vi "onthefly2DfitR4_joe.vi"(0 "Detuning in MHz":dbl=3.1200000000000045, 1 "Wavelength (m)":dbl=4.61e-07, 2 "pass image method":bool=TRUE, 3 "Natural Linewidth of Transition\n(ion fwhm in MHz)":dbl=32.0, 4 "Scale Base Level?":bool, 5 "Systematic Broadening in MHz\n(e.g., 3*naturalwidth)":dbl, 6 "Atoms":sgl[][](array[numeric])=array128x160[20480 elements] format="%0.3f", 10 "Background":sgl[][](array[numeric])=array128x160[20480 elements] format="%0.3f", 12 "Specifics of Fitting Routines":T3={"sampleinterleave"=1.0, "pixelsize"=1.04e-05, "CCDbinning"=1.0, "cutborders"=0.0, "number for scale"=5.0, "limit"=5.0, "guesssmoothsize"=1.0}, 18 "Software bin size":dbl=1.0, 19 "Iteration #":i32=17) -> (7 "2-D Gaussian Fit Parameters":T2={"amplitude"=0.8892961577453615, "sigma_y (m)"=0.0010716344200523828, "sigma_x (m)"=0.0011282187646071032, "row offset (pixel #)"=107.09090196307163, "col offset (pixel #)"=64.60863610301513, "offset"=0.0023484310835031282, "slope x"=3.501893060231643e-06, "slope y"=-1.2386464094312888e-05, 0.0}, 8 "opticaldepthimagesingle\n(ln(atoms)-ln(back))(-1)":dbl[][](graph), 9 "peak OD":dbl=0.8892961577453615, 11 "95% confidence intervals":dbl[][](array[numeric])=[[0.8878200954605137, 0.8907722200302094], [12.85779707503883, 12.902645714681908], [13.536711566357582, 13.583931813620858], [107.06932488748916, 107.1124790386541], [64.585796563439, 64.63147564259125], [0.0021145781066604402, 0.0025822840603458162], [-4.1229500025295996e-07, 7.416081120716245e-06], [-1.707838635719088e-05, -7.694541831434894e-06]], 13 "smoothed OD-fit OD":dbl[][](graph), 14 "# atoms from peakOD":dbl=69475747.95013615 format="%#_6e", 15 "# atoms from \nODintegral":dbl=69475747.95013615, 16 "Chi-squared":dbl=4.589730734027751 format="%#_3g", 17 "alpha":dbl=9.775419954480679e-14)   [LabVIEW 2013]
uses:
  <vilib>/Utility/file.llb/Read From Spreadsheet File (DBL).vi
  <vilib>/Analysis/NI_AALPro.lvlib
panel:
  out "2-D Array of Real":dbl[][](array[numeric])
  in  "Case Constant\n(See Context Help) 3":bool=TRUE
  in  "Case Constant\n(See Context Help) 2":bool=TRUE
  in  "Case Constant\n(See Context Help)":bool
  in  "Read from Binary?":bool=TRUE
  out "Atoms 2":sgl[][](array[numeric])
  out "min index(es)":i32[](array[numeric])=[114, 65]
  out "min value":sgl=98108.0
  out "max index(es)":i32[](array[numeric])=[57, 62]
  out "max value":sgl=690763.0
  out "size(s)":i32[](array[numeric])=[160, 128]
  out "ROI (no binning)":sgl[][](graph)
  out "max indices on\noutput image":i32[](array[numeric])=[96, 56]
  in  "Cut image?":bool
  in  "ROI Controls":T1={"row index"=110, "# rows"=440, "col index"=600, "# cols"=550}
  out "peak indices on\ninput image":i32[](array[numeric])=[96, 56]
  out "error out":errorcluster
  in  "saved image dimensions\n(if saved file is binary)":i32[](array[numeric])=[1024, 1280]
  in  "File Path for image (not background)":path=path "C:/instrumentvi/development/2dfits/20050818atomstestfitB.bny"
  in  "File Path for electronic\nbackground image (must be\nsame size as image of atoms)":path=path "C:/instrumentvi/development/2dfits/20050818backtestfitB.bny"
  out "smoothed optical depth":dbl[][](graph)
  out "fit optical depth":dbl[][](graph)
  out "Background":dbl[][](graph)
  out "Atoms":dbl[][](graph)
  # "Can be gotten\nfrom batch file"
  # "number of columns and rows to scale the base level of atom and background images"
  # "(total column size in each data file should be an integer multiple of sampleinterleave) for big matrices form a matrix using only one point for every sampleinterleave points in a row/column"
  # "the real size for the object in meter unit for a pixel"
  # "number of columns and rows at the corners to find the uncertainities/noise"
  # "total binning"
  # "(REMEMBER THIS IS DONE AFTER SAMPLEINTERLEAVE) number of columns and rows to trim on either side of the data matrix"
  # "number of pixels in smoothing for plotting residuals"
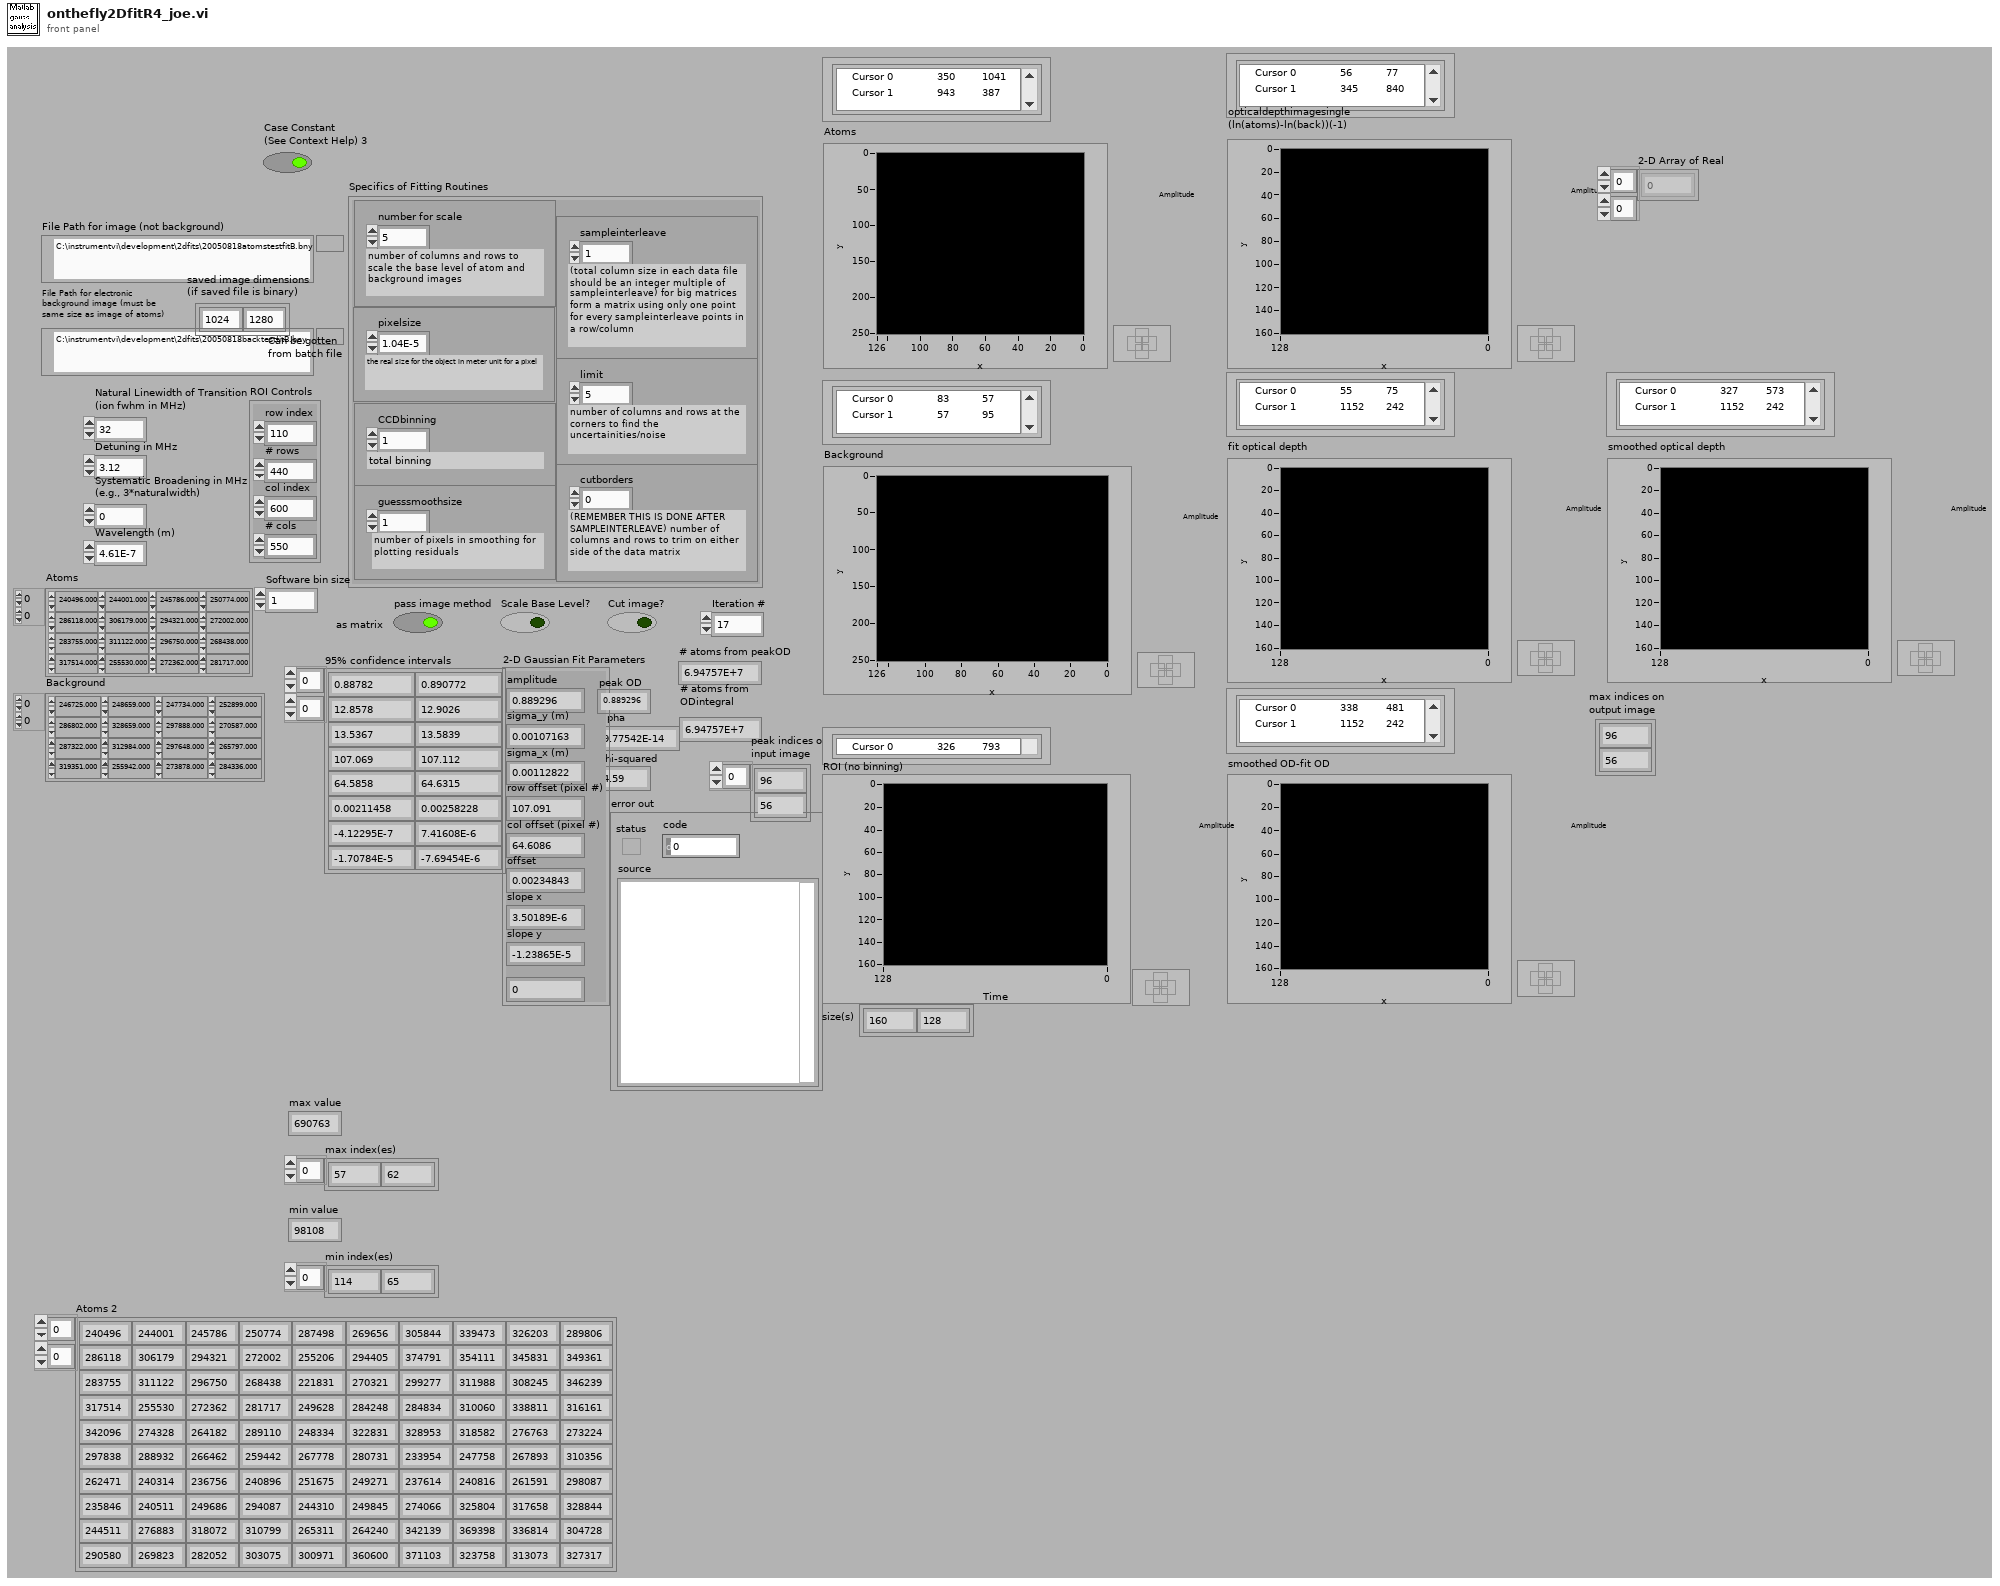
[diagram p1: front panel]
types:
  T1 = cluster{"row index":i32, "# rows":i32, "col index":i32, "# cols":i32}
  T2 = cluster{"amplitude":dbl, "sigma_y (m)":dbl, "sigma_x (m)":dbl, "row offset (pixel #)":dbl, "col offset (pixel #)":dbl, "offset":dbl, "slope x":dbl, "slope y":dbl, dbl}
  T3 = cluster{"sampleinterleave":dbl, "pixelsize":dbl, "CCDbinning":dbl, "cutborders":dbl, "number for scale":dbl, "limit":dbl, "guesssmoothsize":dbl}
  T4 = cluster{"[0]":dbl, "[1]":dbl, "[2]":dbl, "[3]":dbl, "[4]":dbl, "[5]":dbl, "[6]":dbl, "[7]":dbl, "[8]":dbl}
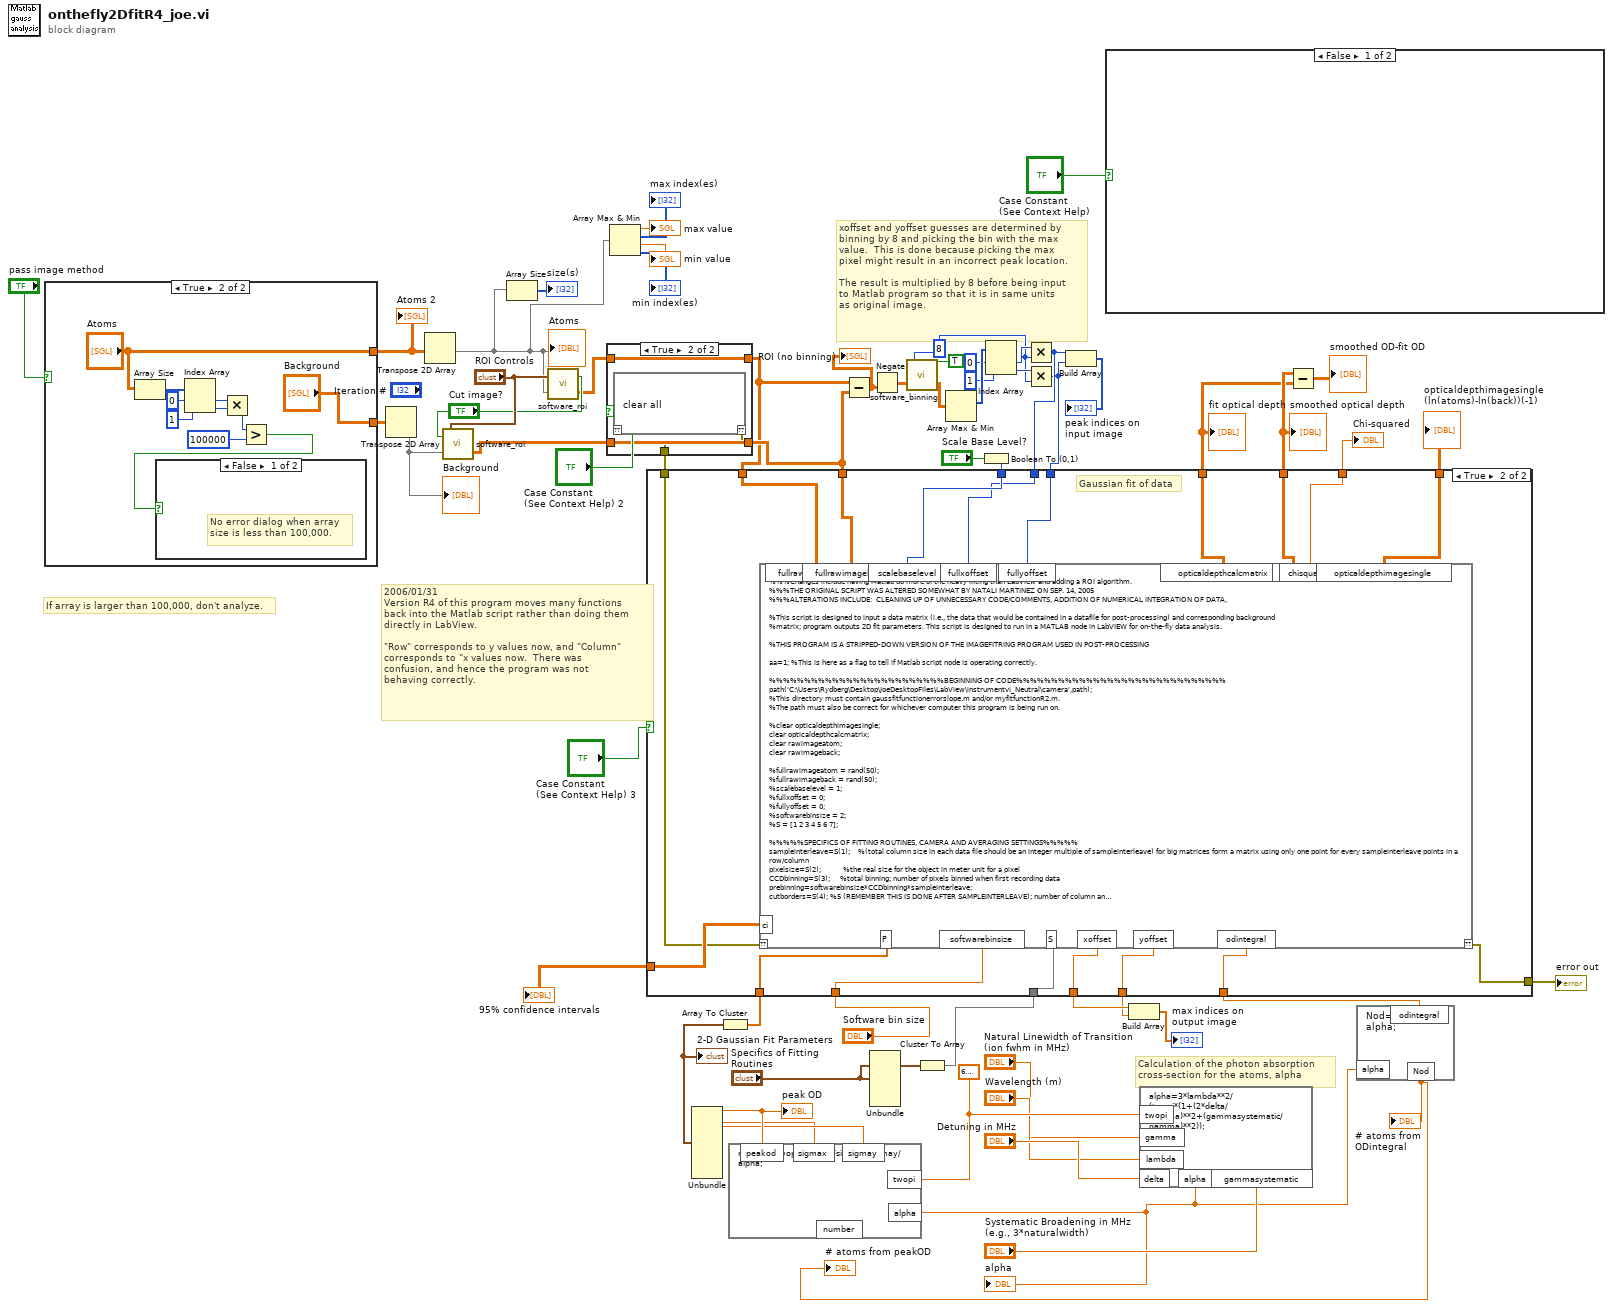
[diagram p0: block diagram]
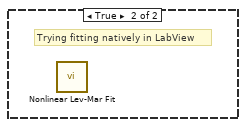
[diagram p2: hidden frame]
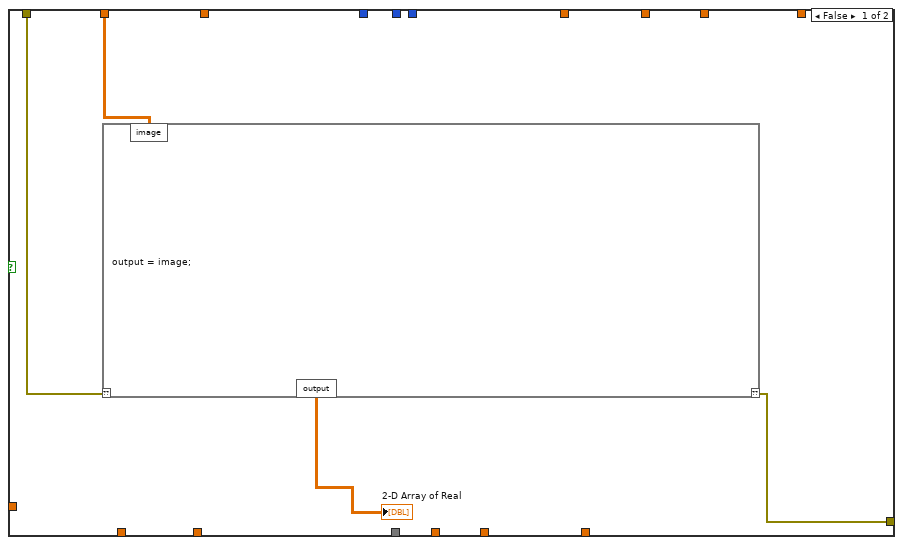
[diagram p3: hidden frame]
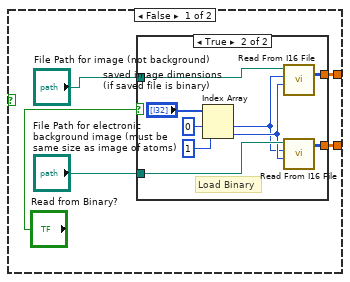
[diagram p5: hidden frame]
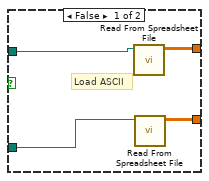
[diagram p6: hidden frame]
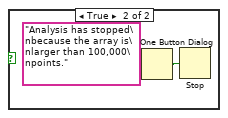
[diagram p7: hidden frame]
diagram:
  w39 = 8 ("bin size")
  w61 = 6.283185307179586
  # "If array is larger than 100,000, don't analyze."
  # "2006/01/31\nVersion R4 of this program moves many functions\nback into the Matlab script rather than doing them\ndirectly in LabView.\n\n\"Row\" corresponds to y values now, and \"Column\"\ncorresponds to \"x values now.  There was\nconfusion, and hence the program was not\nbehaving correctly."
  # "xoffset and yoffset guesses are determined by\nbinning by 8 and picking the bin with the max\nvalue.  This is done because picking the max\npixel might result in an incorrect peak location.\n\nThe result is multiplied by 8 before being input\nto Matlab program so that it is in same units\nas original image."
  # "Calculation of the photon absorption\ncross-section for the atoms, alpha"
  n1 = case shown="True" "pass image method" {
    tunnel: [w66 "Atoms"] -> w16
    tunnel: [w65 "Background"] -> w15
    frame False {
      n2 = case shown="True" "Read from Binary?" {
        tunnel: [w70 w79] -> w66
        tunnel: [w69 w78] -> w65
        tunnel: "File Path for image (not background)" -> [w68 w76]
        tunnel: "File Path for electronic\nbackground image (must be\nsame size as image of atoms)" -> [w67 w77]
        frame False {
          # "Load ASCII"
          n3 = call-poly <vilib>:"Read From Spreadsheet File.vi"("file path (dialog if empty)"=w68) -> ("all rows"=w70:dbl[][])  [unwired: 6 in, 4 out]
          n4 = call-poly <vilib>:"Read From Spreadsheet File.vi"("file path (dialog if empty)"=w67) -> ("all rows"=w69:dbl[][])  [unwired: 6 in, 4 out]
        }
        frame True {
          # "Load Binary"
          n5 = Index Array(array="saved image dimensions\n(if saved file is binary)", index #1=0, index #2=1) -> (element #1=w71:i32, element #2=w72:i32)
          n6 = call <vilib>:"Read From I16 File.vi"("2D number of columns/1D count (all as 1D:-1)"=w72, "2D number of rows"=w71, "file path (dialog if empty)"=w76) -> ("2D array"=w79:i16[][])  [unwired: 4 in, 4 out]
          n7 = call <vilib>:"Read From I16 File.vi"("2D number of columns/1D count (all as 1D:-1)"=w72, "2D number of rows"=w71, "file path (dialog if empty)"=w77) -> ("2D array"=w78:i16[][])  [unwired: 4 in, 4 out]
        }
      }
    }
    frame True {
      n8 = Array Size(array="Atoms") -> (size(s)=w87:i32[])
      n9 = Index Array(array=w87, index #1=0 ("index"), index #2=1 ("index")) -> (element #1=w84:i32, element #2=w83:i32)
      n10 = Multiply(x=w84, y=w83) -> (x*y=w82:i32)
      n11 = Greater?(x=w82, y=100000) -> (0:w80:bool)
      n12 = case shown="False" w80 {
        frame False {
          # "No error dialog when array\nsize is less than 100,000."
        }
        frame True {
          n13 = One Button Dialog(message="Analysis has stopped\nbecause the array is\nlarger than 100,000\npoints.") -> (true=w90:bool)  [unwired: 1 in]
          n14 = Stop(stop? (T)=w90) -> ()
        }
      }
    }
  }
  "Atoms 2" <- w16
  n15 = Transpose 2D Array(2D array=w15) -> (transposed array=w13:dbl[][])
  "Background" <- w13
  n16 = Transpose 2D Array(2D array=w16) -> (transposed array=w10:dbl[][])
  "Atoms" <- w10
  n17 = call "software_roi.vi"("Cut image?"="Cut image?", "Input Array"=w13, "ROI Controls"="ROI Controls") -> ("output array"=w12:sgl[][])
  n18 = Array Size(array=w10) -> (size(s)=→"size(s)":i32[])
  n19 = call "software_roi.vi"("Cut image?"="Cut image?", "Input Array"=w10, "ROI Controls"="ROI Controls") -> ("output array"=w14:sgl[][])
  n20 = case shown="True" "Case Constant\n(See Context Help) 2" {
    tunnel: w14 -> [w93 w96]
    tunnel: [w93 w96] -> w25
    tunnel: [w92 w95] -> w26
    tunnel: w12 -> [w92 w95]
    tunnel: [_ w94] -> w11
    frame False {
    }
    frame True {
      n21 = script code="clear all"() -> ("??"=w94:errorcluster)  [unwired: 1 in]
    }
  }
  n22 = Array Max & Min(array=w10) -> (max value=→"max value":dbl, max index (indices)=→"max index(es)":i32[], min value=→"min value":dbl, min index (indices)=→"min index(es)":i32[])
  n23 = Subtract(x=w25, y=w26) -> (x-y=w18:sgl[][])
  "ROI (no binning)" <- w18
  n24 = Unbundle("Specifics of Fitting Routines") -> ()  [unwired: 7 out]
  n25 = Negate(x=w18) -> (-x=w24:sgl[][])
  n26 = call "software_binning.vi"("Bin image?"=TRUE, "Input Array"=w24, "bin size"=w39) -> ("Binned Array"=w32:dbl[][])
  n27 = Cluster To Array(cluster="Specifics of Fitting Routines") -> (array=w3:dbl[])
  n28 = Array Max & Min(array=w32) -> (max index (indices)=w44:i32[])  [unwired: 3 out]
  n29 = Boolean To (0,1)(Boolean="Scale Base Level?") -> (0, 1=w28:i16)
  n30 = Index Array(array=w44, index #1=0 ("index"), index #2=1 ("index")) -> (element #1=w41:i32, element #2=w40:i32)
  n31 = Multiply(x=w41, y=w39) -> (x*y=w23:i32)
  n32 = Multiply(x=w40, y=w39) -> (x*y=w22:i32)
  n33 = case shown="True" "Case Constant\n(See Context Help) 3" {
    tunnel: [_ w103] -> w60
    tunnel: [_ w109] -> w59
    tunnel: [_ w112] -> w57
    tunnel: [_ w104] -> w48
    tunnel: [w100 w110] -> w1
    tunnel: w25 -> [w98 w102]
    tunnel: w26 -> [_ w118]
    tunnel: [_ w111] -> w27
    tunnel: [_ w114] -> w34
    tunnel: [_ w113] -> w35
    tunnel: w28 -> [_ w117]
    tunnel: w23 -> [_ w116]
    tunnel: w22 -> [_ w115]
    tunnel: [_ w106] -> w21
    tunnel: [_ w105] -> w20
    tunnel: w11 -> [w99 w101]
    tunnel: w3 -> [_ w107]
    tunnel: "Software bin size" -> [_ w108]
    frame False {
      n34 = script code="output = image;"("??"=w99, "image"=w98) -> ("??"=w100:errorcluster, "output"=→"2-D Array of Real":dbl[][])
    }
    frame True {
      # "Gaussian fit of data"
      n35 = script code="%%%Last revision 2006/01/30, by Pascal.\n%%%Changes include having Matlab do more of the heavy lifting than LabView and adding a ROI algorithm.\n%%%THE ORIGINAL SCRIPT WAS ALTERED SOMEWHAT BY NATALI MARTINEZ ON SEP. 14, 2005\n%%%ALTERATIONS INCLUDE:  CLEANING UP OF UNNECESSARY CODE/COMMENTS, ADDITION OF NUMERICAL INTEGRATION OF DATA,  \n\n%This script is designed to input a data matrix (i.e., the data that would be contained in a datafile for post-processing) and corresponding background \n%matrix; program outputs 2D fit parameters. This script is designed to run in a MATLAB node in LabVIEW for on-the-fly data analysis.\n\n%THIS PROGRAM IS A STRIPPED-DOWN VERSION OF THE IMAGEFITRING PROGRAM USED IN POST-PROCESSING\n\naa=1; %This is here as a flag to tell if Matlab script node is operating correctly.\n\n%%%%%%%%%%%%%%%%%%%%%%%%%BEGINNING OF CODE%%%%%%%%%%%%%%%%%%%%%%%%%%%%%%\npath('C:\\Users\\Rydberg\\Desktop\\JoeDesktopFiles\\LabView\\instrumentvi_Neutral\\camera',path);\n%This directory must contain gaussfitfunctionerrorslope.m and/or myfitfunctionR2.m.\n%The path must also be correct for whichever computer this program is being run on.\n\n%clear opticaldepthimagesingle;\nclear opticaldepthcalcmatrix;\nclear rawimageatom;\nclear rawimageback;\n\n%fullrawimageatom = rand(50);\n%fullrawimageback = rand(50);\n%scalebaselevel = 1;\n%fullxoffset = 0;\n%fullyoffset = 0;\n%softwarebinsize = 2;\n%S = [1 2 3 4 5 6 7];\n\n%%%%%SPECIFICS OF FITTING ROUTINES, CAMERA AND AVERAGING SETTINGS%%%%%\nsampleinterleave=S(1);    %(total column size in each data file should be an integer multiple of sampleinterleave) for big matrices form a matrix using only one point for every sampleinterleave points in a row/column\npixelsize=S(2);           %the real size for the object in meter unit for a pixel\nCCDbinning=S(3);     %total binning; number of pixels binned when first recording data\nprebinning=softwarebinsize*CCDbinning*sampleinterleave;\ncutborders=S(4); %5 (REMEMBER THIS IS DONE AFTER SAMPLEINTERLEAVE); number of column and rows to trim on either side of the data matrix\nnumberforscale=S(5);     %number of column and rows to scale the base level of atom and background images\nlimit=S(6);     %number of column and rows at the corners to find the uncertainities/noise\nguesssmoothsize=S(7);  %number of points to average for guessing\n\nf=fullrawimageatom;\nfullsizefull=size(fullrawimageatom);\nfullrowfull=fullsizefull(1); %no. of rows; form matrix from only part of the data\nfullcolumnfull=fullsizefull(2);\n\n%%%SCALING OF BASE LEVEL%%%\nif scalebaselevel==1\n     sumylowxlow=sum(sum(fullrawimageatom(1:numberforscale,1:numberforscale)));;\n     sumylowxhigh=sum(sum(fullrawimageatom(1:numberforscale,fullcolumnfull-numberforscale:fullcolumnfull)));\n     sumyhighxlow=sum(sum(fullrawimageatom(fullrowfull-numberforscale:fullrowfull,1:numberforscale)));\n     sumyhighxhigh=sum(sum(fullrawimageatom(fullrowfull-numberforscale:fullrowfull,fullcolumnfull-numberforscale:fullcolumnfull)));\n     baselevelatom=sumylowxlow+sumylowxhigh+sumyhighxlow+sumyhighxhigh;\n     sumylowxlow=sum(sum(fullrawimageback(1:numberforscale,1:numberforscale))); %there was an error I think so changed from average to sum since \n     sumylowxhigh=sum(sum(fullrawimageback(1:numberforscale,fullcolumnfull-numberforscale:fullcolumnfull)));\n     sumyhighxlow=sum(sum(fullrawimageback(fullrowfull-numberforscale:fullrowfull,1:numberforscale)));\n     sumyhighxhigh=sum(sum(fullrawimageback(fullrowfull-numberforscale:fullrowfull,fullcolumnfull-numberforscale:fullcolumnfull)));\n     baselevelback=sumylowxlow+sumylowxhigh+sumyhighxlow+sumyhighxhigh;\n     fullrawimageatom=fullrawimageatom*baselevelback/baselevelatom;\nend\n\n%%%INTERLEAVING OF DATA%%%;  uses every sampleinterleave points and throws away rest of data\ni=0; j=0; v=0;\nfor i=1:fullrowfull/sampleinterleave\n    for j=1:fullcolumnfull/sampleinterleave\n        for v=1:sampleinterleave\n            temp1(v)=sum(fullrawimageatom(((i-1)*sampleinterleave+1):i*sampleinterleave,((j-1)*sampleinterleave+v))); %this does the software interleaving/sampling\n            temp2(v)=sum(fullrawimageback(((i-1)*sampleinterleave+1):i*sampleinterleave,((j-1)*sampleinterleave+v))); %interleaving for background\n        end\n        rawimageatom(i,j)=sum(temp1); %stores the software interleaved/sampled data\n        rawimageback(i,j)=sum(temp2); %stores the software interleaved/sampled data\n    end\nend\nsizefull=size(rawimageatom);\nrowfull=sizefull(1);       %number of rows after interleaving\ncolumnfull=sizefull(2); %number of columns after interleaving\nxoffsetfull=fullxoffset/sampleinterleave; %adjust peak position to new size\nyoffsetfull=fullyoffset/sampleinterleave; %adjust peak position to new size\n\n%%%CUT DATA OFF FROM EDGES%%%; remember this is done after interleaving\ni=0; j=0;\nfor i=1+cutborders:rowfull-cutborders,\n    for j=1+cutborders:columnfull-cutborders,\n        cutimageatom(i-cutborders,j-cutborders)=rawimageatom(i,j);\n        cutimageback(i-cutborders,j-cutborders)=rawimageback(i,j);\n    end\nend\nsizes=size(cutimageatom);\nrow=sizes(1); %number of rows after cutting data off of edges\ncolumn=sizes(2); %number of columns after cutting data off of edges\nxoffset=xoffsetfull-cutborders; %Determines guess for peak position\nyoffset=yoffsetfull-cutborders; %Determines guess for peak position\n\n%%%ABS VALUE AND OPTICAL DEPTH%%%\ncutimageatom=abs(cutimageatom);   %abs gives the absolute value and complex magnitude\ncutimageback=abs(cutimageback);\nopticaldepthimagesingle=(log(cutimageatom)-log(cutimageback))*(-1); %makes absorption positive\n\n%%%DATA FITTING - 2D FITS%%%\n%GENERATE GUESSES AND BOUNDS%\nZguess=filter2(ones(guesssmoothsize,guesssmoothsize),opticaldepthimagesingle(:,:))/guesssmoothsize^2; %atom-back/OD, smoothed for finding guesses   \namplitude=max(max(Zguess));     %this will give trouble if slope is too big\nsigx=column/10;\nsigy=row/10;\n%xoffset=row/2; %xoffset is now input from LabView; determined by binning by 8 and choosing max bin rather than max pixel.\n%yoffset=column/2; %same comment for yoffset as for xoffset.\naverageylowxlow=sum(sum(Zguess(1:5,1:5)))/25;;\naverageylowxhigh=sum(sum(Zguess(1:5,column-5:column)))/25;\naverageyhighxlow=sum(sum(Zguess(row-5:row,1:5)))/25;\naverageyhighxhigh=sum(sum(Zguess(row-5:row,column-5:column)))/25;\noffset=(averageylowxlow+averageylowxhigh+averageyhighxlow+averageyhighxhigh)/4 ;\nslopex=((averageylowxhigh+averageyhighxhigh)-(averageylowxlow+averageyhighxlow))/(2*column);\nslopey=((averageyhighxlow+averageyhighxhigh)-(averageylowxlow+averageylowxhigh))/(2*row);\n     \nInitialConditions=[amplitude, sigx, sigy, xoffset, yoffset,offset,slopex,slopey];\n%lowerbound=[0, 1, 1, 10, 10, -3, 0, 0,-.01,-.01];\n%upperbound=[1, 50, 50, 90, 90, 3, 1, 1,.01,.01];\ntemp5=size(InitialConditions);\nnumberofparameters=temp5(2); %number of 2D fit parameters\n \n%%%STATISTICS OF IMAGE%%%\n%Weird things happen when you calculate these with smoothed images!!!\n%get estimate of noise, you need to subtract image from background because of fringes and variations in intensity\naverage1=sum(sum(cutimageatom(1:limit,1:limit)-cutimageback(1:limit,1:limit)))/limit^2;\nrms1=sqrt(sum(sum((cutimageatom(1:limit,1:limit)-cutimageback(1:limit,1:limit)).^2))/limit^2);\nrmsdeviation1=sqrt(rms1^2-average1^2);\n   \naverage2=sum(sum(cutimageatom(row-limit:row,1:limit)-cutimageback(row-limit:row,1:limit)))/limit^2;\nrms2=sqrt(sum(sum((cutimageatom(row-limit:row,1:limit)-cutimageback(row-limit:row,1:limit)).^2))/limit^2);\nrmsdeviation2=sqrt(rms2^2-average2^2);\n   \naverage3=sum(sum(cutimageatom(1:limit,column-limit:column)-cutimageback(1:limit,column-limit:column)))/limit^2;\nrms3=sqrt(sum(sum((cutimageatom(1:limit,column-limit:column)-cutimageback(1:limit,column-limit:column)).^2))/limit^2);\nrmsdeviation3=sqrt(rms3^2-average3^2);\n\naverage4=sum(sum(cutimageatom(row-limit:row,column-limit:column)-cutimageback(row-limit:row,column-limit:column)))/limit^2;\nrms4=sqrt(sum(sum((cutimageatom(row-limit:row,column-limit:column)-cutimageback(row-limit:row,column-limit:column)).^2))/limit^2);\nrmsdeviation4=sqrt(rms4^2-average4^2);\n   \nerror=abs((rmsdeviation1+rmsdeviation2+rmsdeviation3+rmsdeviation4)/(4))\n\n%%%CREATE FITTING MATRICES%%%\n%SEE EXPLANATION ON PG. 78 OF PRIYA'S NOTEBOOK 2 %\nerrorod(1:row*column)=error/(sum(sum(cutimageback))/(row*column));     %normalized error - relative to average pixel value\nxvec=1:column;\nyvec=1:row;\n[ydata,xdata]=meshgrid(yvec,xvec);     %rows of output array xdata are copies of vector xvec; columns of output array ydata are copies of vector yvec\nydata=transpose(ydata); xdata=transpose(xdata);\nnumberofpoints=column*row*ones(column,row);     %matrix in which each entry is the number of points \ncoordmatrix=[ydata(:),xdata(:),errorod(:),numberofpoints(:)];\n \n%%%ACTUAL FITTING PROCEDURES%%%  \nZ2=(opticaldepthimagesingle(:)./(errorod(:)*sqrt(column*row)));     %flattened(1D) list of image weighted by uncertainties, not smoothed\noptions=statset('MaxIter',12);\n\n%%%nlinfit method%%%\n[P,r,J,iteractual]=nlinfit(coordmatrix,Z2(:),@gaussfitfunctionerrorsslope,InitialConditions,options);     % expecting data divided by weight and sqrt(number of points)\n\n%%%Gauss-Newton least squares%%%\n%maxiter = 10;\n%tol = 10e-5;\n%P = InitialConditions';\n    %for iter = 1:maxiter\n        %[r,J] = feval(@myfitfunctionR2,P,coordmatrix,Z2);\n        %g = J'*r;\n        %nrmg = norm(g);\n        %fprintf('iter: %2i  norm(g) = %7.3e\\n',iter,nrmg);\n        %if nrmg < tol break; end\n\n        %f = 0.5*r'*r;\n        %B = J'*J+min(10e-4,2*f)*speye(size(J,2));\n        %P = P - B\\g;\n    %end\n%P=P';\n\n%%%REMOVE THE GRADIENT FROM THE DATA%%% ; that is, remove background and slope from data\ngradmatrix=(ydata(:)-P(5))*P(8)+(xdata(:)-P(4))*P(7)+P(6);\nnogradoddata=opticaldepthimagesingle(:)-gradmatrix(:);\nnogradodmatrix = reshape(nogradoddata, size(ydata));  %returns an n-dimensional array with same elements as nograddata but reshaped to size(ydata)\n\n%%%Generate plot of optical density based on fitted parameters, remove distortion of data due to dividing by weight and sqrt(number of points)%%%\ndummyerrorod(1:row*column)=1; \ndummynumberofpoints=ones(row,column); \ncoordmatrix=[ydata(:),xdata(:),dummyerrorod(:),dummynumberofpoints(:)];\nopticaldepthcalcvector=gaussfitfunctionerrorsslope(P, coordmatrix);     %optical depth calculated from fit paramters\nopticaldepthcalcmatrix=reshape(opticaldepthcalcvector,size(ydata));\n\nci=nlparci(P,r,J);%error in the fit parameters 95% confidence interval\nsdev=(ci(:,2)-ci(:,1))/4;%turn confidence interval into 1 sigma             \nweightedresidue3D=(Z2(:)-gaussfitfunctionerrorsslope(P, coordmatrix)); %weighted residues\nchi3D=(transpose(weightedresidue3D)*weightedresidue3D)\n%%%CALCULATE CHI-SQUARED%%%\nchisquared=sum(sum((opticaldepthimagesingle-opticaldepthcalcmatrix).*(opticaldepthimagesingle-opticaldepthcalcmatrix)))/((row*column-1)*errorod(1)^2);\n%Fraction absorption is p(1)\n\n%%%CALCULATING OD INTEGRAL%%%\ntotalod=0;\nodintegral=0;\n%%%Sum of the optical depth to get the total OD%%%\ni=0; j=0; pixelcount=0;\nfor i=1:row\n     for j=1:column\n          tempindex=(i-1).*column+j; %converts the 2-D index to 1-D so reads from beginning of first row then from beginning of second row and so on\n          totalod=totalod+nogradoddata(tempindex);\n          pixelcount=pixelcount+1;\n     end\nend\n\nodintegral=totalod*(prebinning*pixelsize)^2; %convert to real units, take care of binning effects, etc\nodintegralerror=errorod(1)*sqrt(row*column)*(prebinning*pixelsize)^2;\n\n%%%OUTPUT PARAMETERS%%%\n%These are actually output as P, but names left in so they can be checked in Matlab more easily.\npeakod=P(1);\nP(2)=pixelsize*prebinning*abs(P(2));     %sigmax in meters\nP(3)=pixelsize*prebinning*abs(P(3));     %sigmay in meters\nxcenter=P(4); %xoffset\nycenter=P(5); %yoffset\noffsetfit=P(6);\n\n%%%THE END%%%"("??"=w101, "fullrawimageatom"=w102, "fullrawimageback"=w118, "scalebaselevel"=w117, "fullxoffset"=w116, "fullyoffset"=w115, "softwarebinsize"=w108, "S"=w107) -> ("??"=w110:errorcluster, "opticaldepthcalcmatrix"=w114:dbl[][], "Zguess"=w113:dbl[][], "chisquared"=w112:dbl, "opticaldepthimagesingle"=w111:dbl[][], "ci"=w103:dbl[][], "P"=w109:dbl[], "xoffset"=w106:dbl, "yoffset"=w105:dbl, "odintegral"=w104:dbl)
    }
  }
  "95% confidence intervals" <- w60
  "Chi-squared" <- w57
  "fit optical depth" <- w34
  "smoothed optical depth" <- w35
  "error out" <- w1
  "opticaldepthimagesingle\n(ln(atoms)-ln(back))(-1)" <- w27
  n36 = Array To Cluster(array=w59) -> (cluster=w30:T4)
  "2-D Gaussian Fit Parameters" <- w30
  n37 = Unbundle(w30) -> ("[0]"=w58:dbl, "[1]"=w49:dbl, "[2]"=w50:dbl)  [unwired: 6 out]
  "peak OD" <- w58
  n38 = Build Array(w23, w22) -> (→"peak indices on\ninput image":i32[])
  n39 = case shown="False" "Case Constant\n(See Context Help)" {
    frame False {
    }
    frame True {
      # "Trying fitting natively in LabView"
      n40 = call <vilib>:"Nonlinear Lev-Mar Fit.vi"() -> ()  [unwired: 6 in, 5 out]
    }
  }
  n41 = Build Array(w21, w20) -> (→"max indices on\noutput image":dbl[])
  n42 = formula code="alpha=3*lambda**2/(twopi*(1+(2*delta/gamma)**2+(gammasystematic/gamma)**2));"("delta"="Detuning in MHz", "gamma"="Natural Linewidth of Transition\n(ion fwhm in MHz)", "twopi"=w61, "lambda"="Wavelength (m)", "gammasystematic"="Systematic Broadening in MHz\n(e.g., 3*naturalwidth)") -> ("alpha"=w47:dbl)
  "alpha" <- w47
  n43 = formula code="number=twopi*peakod*sigmax*sigmay/alpha;"("twopi"=w61, "sigmax"=w49, "sigmay"=w50, "peakod"=w58, "alpha"=w47) -> ()  [unwired: 1 out]
  n44 = Subtract(x=w35, y=w34) -> (x-y=→"smoothed OD-fit OD":dbl[][])
  n45 = formula code="Nod=odintegral/alpha;"("odintegral"=w48, "alpha"=w47) -> ("Nod"=→"# atoms from peakOD" →"# atoms from \nODintegral":dbl)
